vi "Get Model Construction.vi"(1 "panel record":string[](array[string])) -> (0 "Fabric Array":string[][](array[string]))   [LabVIEW 2015]
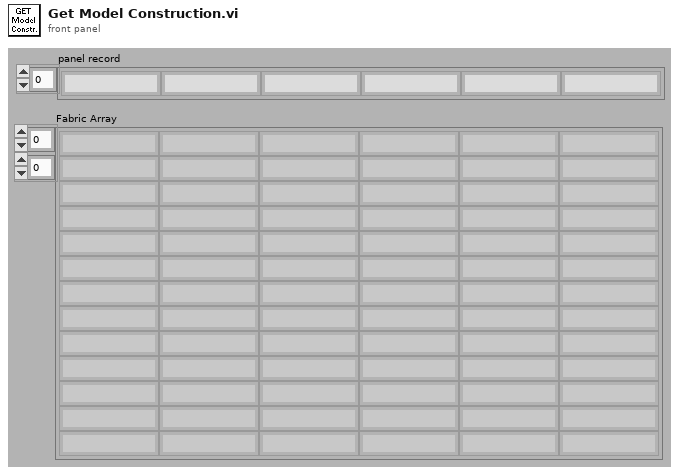
[diagram p1: front panel]
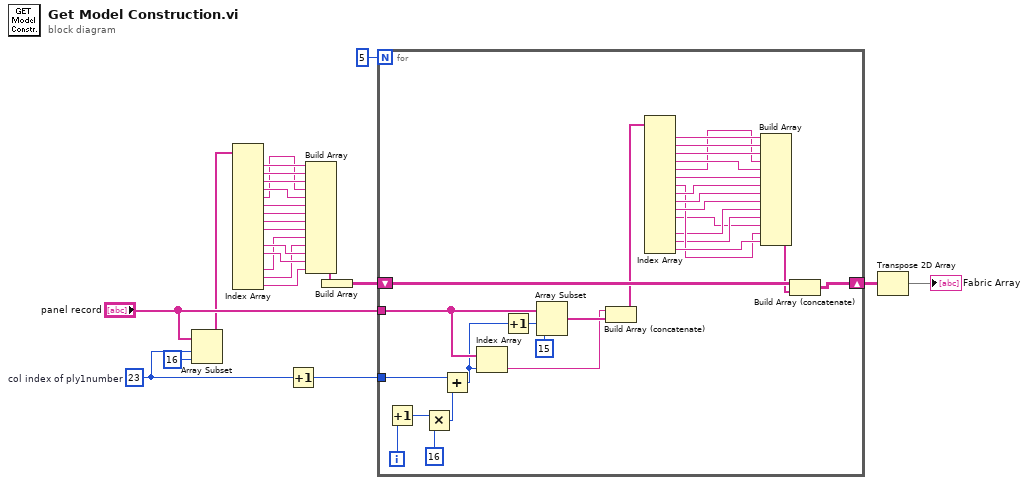
[diagram p0: block diagram]
diagram:
  w23 = 23  # col index of ply1number
  n1 = Array Subset(array="panel record", index=w23, length=16) -> (w15:string[])
  n2 = Index Array(array=w15) -> (element #1=w7:string, element #2=w17:string, element #3=w16:string, element #4=w2:string, element #5=w1:string, element #6=w14:string, element #7=w13:string, element #8=w12:string, element #9=w11:string, element #11=w10:string, element #12=w9:string, element #14=w4:string, element #15=w5:string, element #16=w6:string)  [unwired: 16 in, 2 out]
  n3 = Increment(x=w23) -> (x+1=w3:i32)
  n4 = Build Array(w7, w17, w16, w1, w2, w14, w13, w12, w11, w4, w5, w10, w9, w6) -> (w8:string[])
  n5 = Build Array(w8) -> (w22:string[][])
  n6 = for {
    N: 5 -> [_]
    shift-right: [w52] -> w20
    shift-left: w22 -> [w53]
    tunnel: "panel record" -> [w46]
    tunnel: w3 -> [w51]
    i -> [w50]
    n7 = Increment(x=w50) -> (x+1=w47:i32)
    n8 = Multiply(x=w47, y=16) -> (x*y=w48:i32)
    n9 = Add(x=w51, y=w48) -> (x+y=w45:i32)
    n10 = Index Array(array=w46, index=w45) -> (element=w41:string)
    n11 = Increment(x=w45) -> (x+1=w43:i32)
    n12 = Array Subset(array=w46, index=w43, length=15) -> (w44:string[])
    n13 = Build Array (concatenate)(w41, w44) -> (w36:string[])
    n14 = Index Array(array=w36) -> (element #1=w40:string, element #2=w37:string, element #3=w38:string, element #4=w26:string, element #5=w25:string, element #6=w39:string, element #7=w30:string, element #8=w34:string, element #9=w33:string, element #10=w32:string, element #11=w27:string, element #13=w29:string, element #14=w28:string, element #15=w31:string)  [unwired: 15 in, 1 out]
    n15 = Build Array(w40, w37, w38, w25, w26, w39, w34, w33, w32, w29, w28, w27, w30, w31) -> (w35:string[])
    n16 = Build Array (concatenate)(w53, w35) -> (w52:string[][])
  }
  n17 = Transpose 2D Array(2D array=w20) -> (transposed array=→"Fabric Array":string[][])
